vi "PiezoGetPosition.vi"(4 "error in (no error)":errorcluster, 7 "reference":refnum<k7>) -> (0 "error out":errorcluster, 2 "Position":sgl, 3 "reference out":refnum<k7>)   [LabVIEW 2018]
uses:
  <userlib>/bpc203/PiezoChannelNumber.ctl
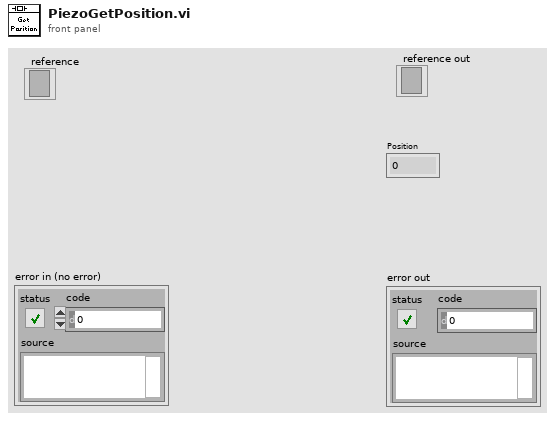
[diagram p1: front panel]
types:
  T1 = typedef "PiezoChannelNumber.ctl" = u16
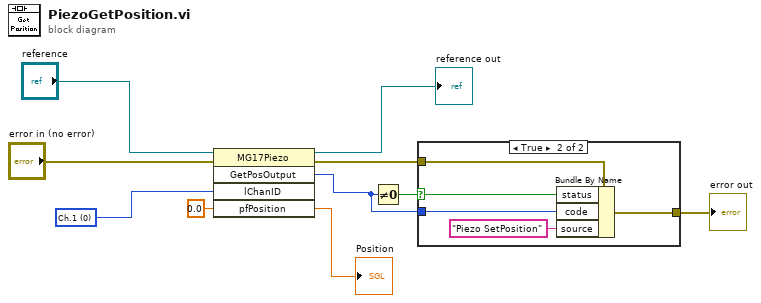
[diagram p0: block diagram]
diagram:
  w8 = T1 0 items=["Ch.1", "Ch.2"] ("lChanID")
  n1 = invoke class="MG17Piezo" method="GetPosOutput"(reference="reference", error in="error in (no error)", "lChanID"=w8, "pfPosition"=sgl 0.0) -> (reference out=→"reference out":refnum<k7>, error out=w5:errorcluster, "GetPosOutput"=w3:i32, "pfPosition"=→"Position":sgl)  [unwired: 1 in, 1 out]
  n2 = Not Equal To 0?(x=w3) -> (x != 0?=w6:bool)
  n3 = case shown="True" w6 {
    selector: w6 -> [_ w15]
    tunnel: w5 -> [w11 w16]
    tunnel: [w11 w13] -> w4
    tunnel: w3 -> [_ w12]
    frame False {
    }
    frame True {
      n4 = Bundle By Name(cluster=w16, "status"=w15, "code"=w12, "source"="Piezo SetPosition") -> (w13:errorcluster)
    }
  }
  "error out" <- w4
